vi "Ball Viewer.vi"(11 "balls":T1[](array[typedef])) -> ()   [LabVIEW 2016]
uses:
  SSL Detection Ball.ctl
  <vilib>/Analysis/Matrix/Datatypes/RealMatrix.ctl
  <vilib>/Analysis/Matrix/NI_Matrix.lvlib
panel:
  out "Waveform Chart":dbl(graph)
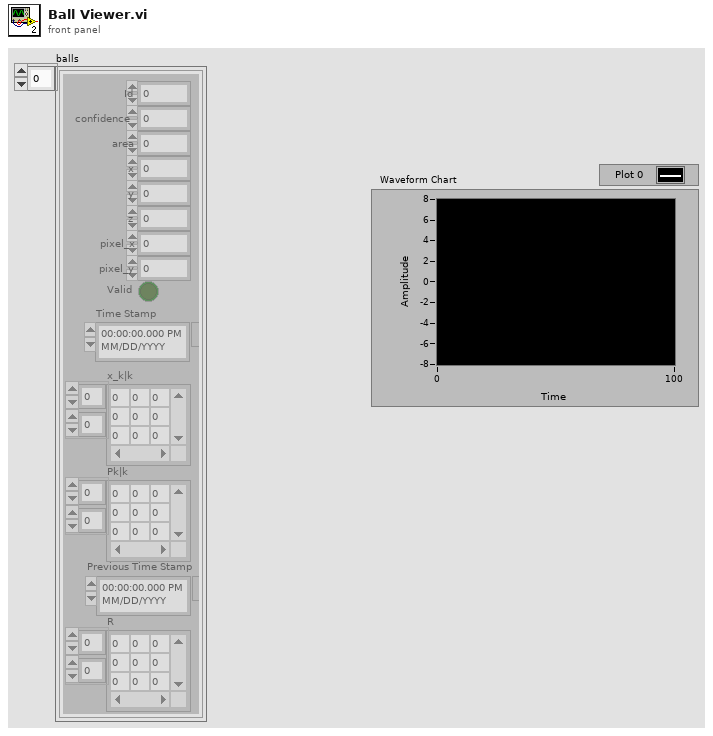
[diagram p1: front panel]
types:
  T1 = typedef "SSL Detection Ball.ctl" = cluster{"x":sgl, "area":u32, "confidence":sgl, "y":sgl, "z":sgl, "pixel_x":sgl, "pixel_y":sgl, "Valid":bool, "Time Stamp":timestamp, "x_k|k":T2, "Pk|k":T2, "Id":u32, "Previous Time Stamp":timestamp, "R":T2}
  T2 = typedef "NI_Matrix.lvlib/RealMatrix.ctl" = dbl[][]
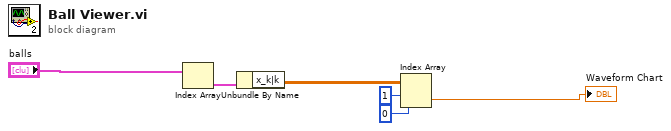
[diagram p0: block diagram]
diagram:
  n1 = Index Array(array="balls") -> (element=w3:T1)  [unwired: 1 in]
  n2 = Unbundle By Name(w3) -> ("x_k|k"=w4:T2)
  n3 = Index Array(array=w4, index (row)=1, index (col)=0 ("disabled index (col)")) -> (element=→"Waveform Chart":dbl)
